vi "Requst Data Control.vi"(11 "Initial address counter":u32) -> (3 "Enable request":bool)   [LabVIEW 2015]
uses:
  <vilib>/rvi/Emulation/niFpgaSctlEmulationGetInTimedLoop.vi
  OpenScan Labview code_20170126/Global_Sample per Frame.vi
  <vilib>/rvi/Emulation/niFpgaProcessEmulError.vi
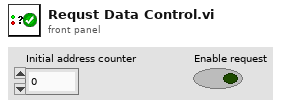
[diagram p1: front panel]
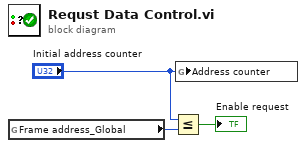
[diagram p0: block diagram]
diagram:
  n1 = global read "Global_Sample per Frame.vi" "Frame address_Global"() -> (w2:u32)
  n2 = Less Or Equal?(x="Initial address counter", y=w2) -> (x <= y?=→"Enable request":bool)
  n3 = global write "Global_Sample per Frame.vi" "Address counter"("Initial address counter") -> ()
